vi "Write_Parameter_To_Data_Packet.vi"(8 "error in (no error)":errorcluster, 10 "Parameter value":string, 11 "Parameter name":string) -> (0 "error out":errorcluster, 3 "Data Packets Out":T1[](array[typedef]))   [LabVIEW 2017]
uses:
  Controls/Data Packets/Data_Packet.ctl
  Controls/Packet/Packet.ctl
  Controls/Packet/Packet_Direction.ctl
  Controls/Packet/Packet_Type.ctl
  Controls/Packet/Packet_Priority.ctl
  Controls/Data Packets/Parameter.ctl
  Controls/Data Packets/Parameter_Data_Type.ctl
  Controls/Data Packets/Data_Packet_Transmit_Mode.ctl
  Controls/Data Packets/Data_Packet_FGV_Commands.ctl
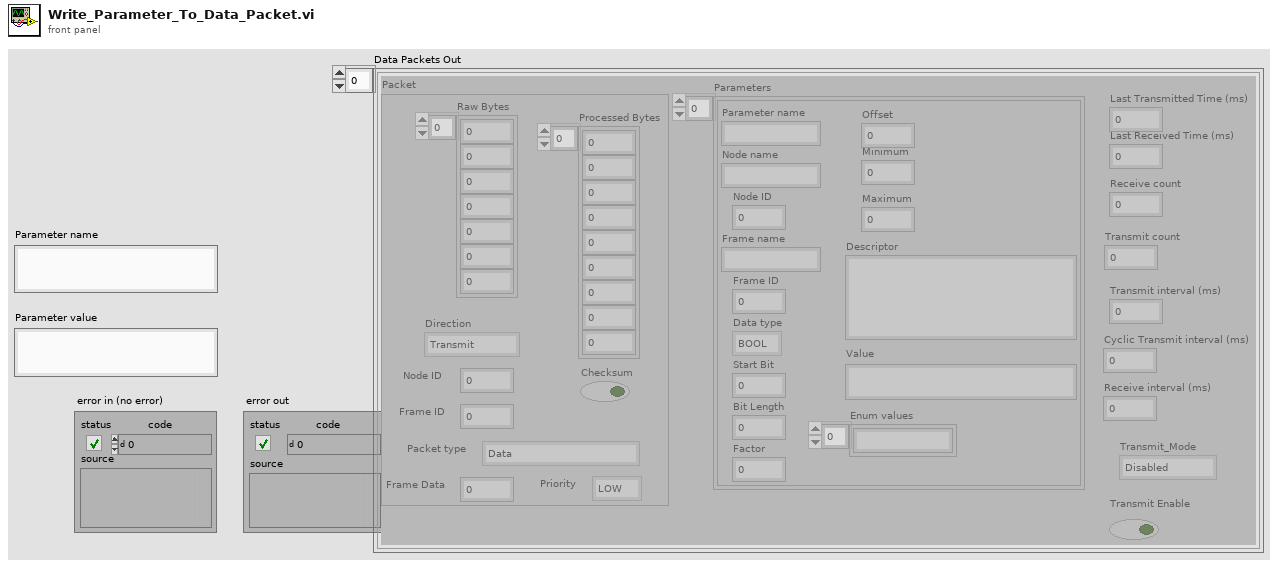
[diagram p1: front panel]
types:
  T1 = typedef "Data_Packet.ctl" = cluster{"Packet":T2, "Parameters":T6[], "Last Received Time (ms)":u64, "Receive count":i32, "Transmit count":i32, "Transmit interval (ms)":u32, "Last Transmitted Time (ms)":u64, "Receive interval (ms)":u32, "Transmit_Mode":T8, "Transmit Enable":bool, "Cyclic Transmit interval (ms)":u32}
  T2 = typedef "Packet.ctl" = cluster{"Raw Bytes":u8[], "Checksum":bool, "Direction":T3, "Processed Bytes":u8[], "Node ID":u8, "Packet type":T4, "Frame Data":u32, "Priority":T5, "Frame ID":u8}
  T3 = typedef "Packet_Direction.ctl" = enum16{"Transmit", "Receive", "Bidirectional"}
  T4 = typedef "Packet_Type.ctl" = enum16{"Data", "Connection Management", "Remote Request", "Error/Status"}
  T5 = typedef "Packet_Priority.ctl" = enum16{"LOW", "HIGH"}
  T6 = typedef "Parameter.ctl" = cluster{"Parameter name":string, "Node name":string, "Node ID":u8, "Frame name":string, "Frame ID":u8, "Data type":T7, "Start Bit":i32, "Bit Length":i32, "Factor":dbl, "Offset":dbl, "Minimum":dbl, "Maximum":dbl, "Descriptor":string, "Enum values":string[], "Value":string}
  T7 = typedef "Parameter_Data_Type.ctl" = enum16{"BOOL", "UNSIGNED", "SIGNED", "FLOAT32", "ENUM"}
  T8 = typedef "Data_Packet_Transmit_Mode.ctl" = enum16{"Disabled", "Single", "Cyclic"}
  T9 = typedef "Data_Packet_FGV_Commands.ctl" = enum16{"Update all parameters from data packets", "Update Packet", "Load", "Read Packet Parameters", "Write Packet Parameters", "Read Packet Parameter", "Write Packet Parameter", "Read Data Packets", "Read Data Packet", "Read Data Packet by Parameter Name", "Get Parameter Node and Frame ID", "Read Data Packet from Node ID and Frame ID"}
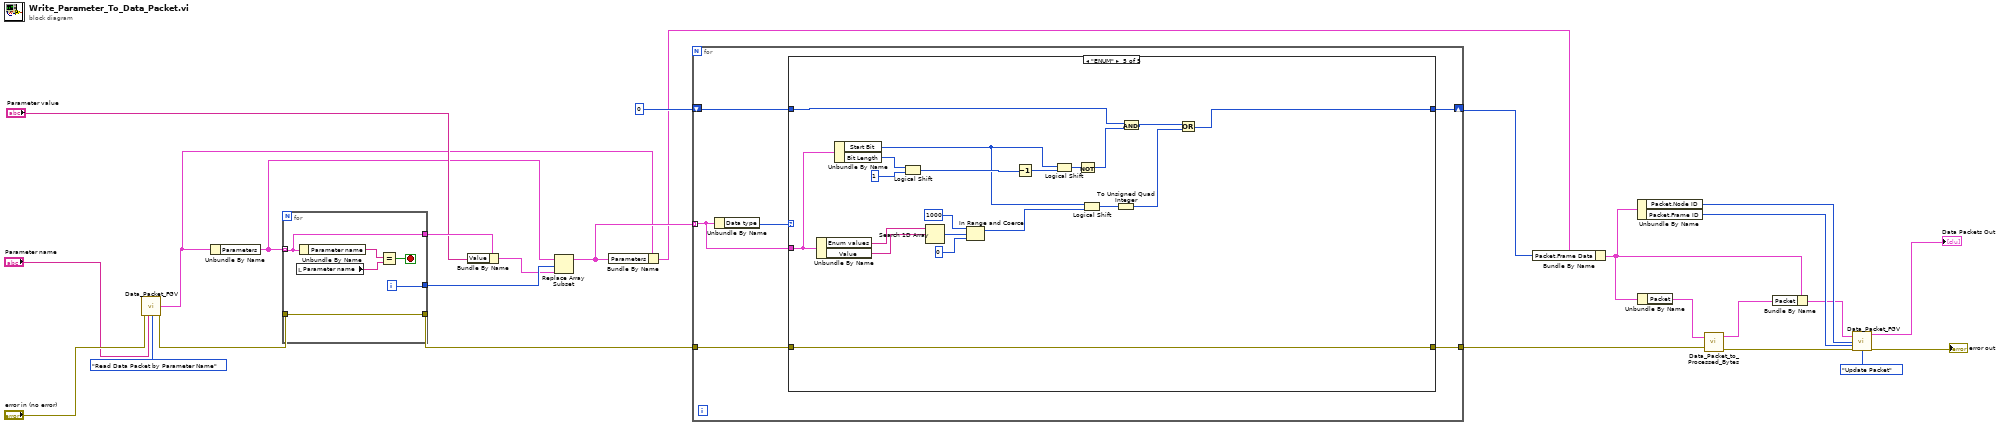
[diagram p0: block diagram]
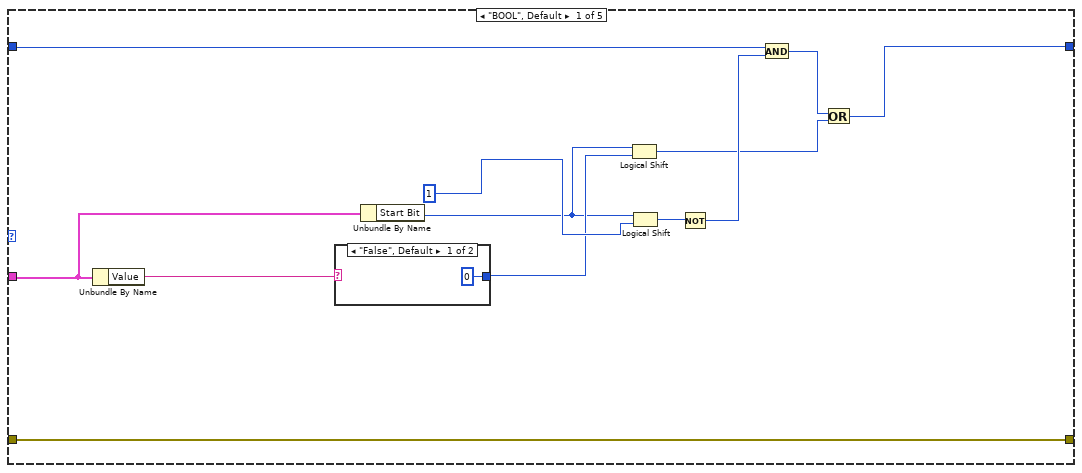
[diagram p2: hidden frame]
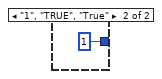
[diagram p3: hidden frame]
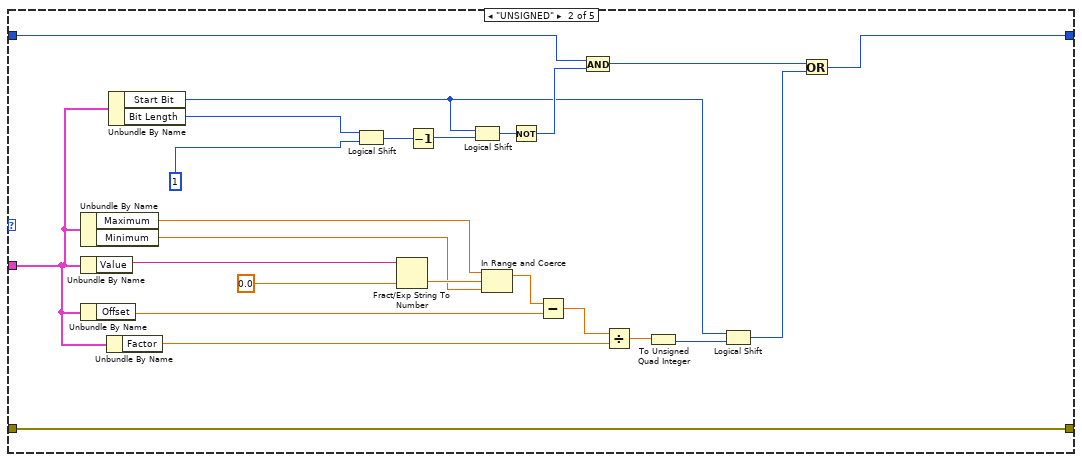
[diagram p4: hidden frame]
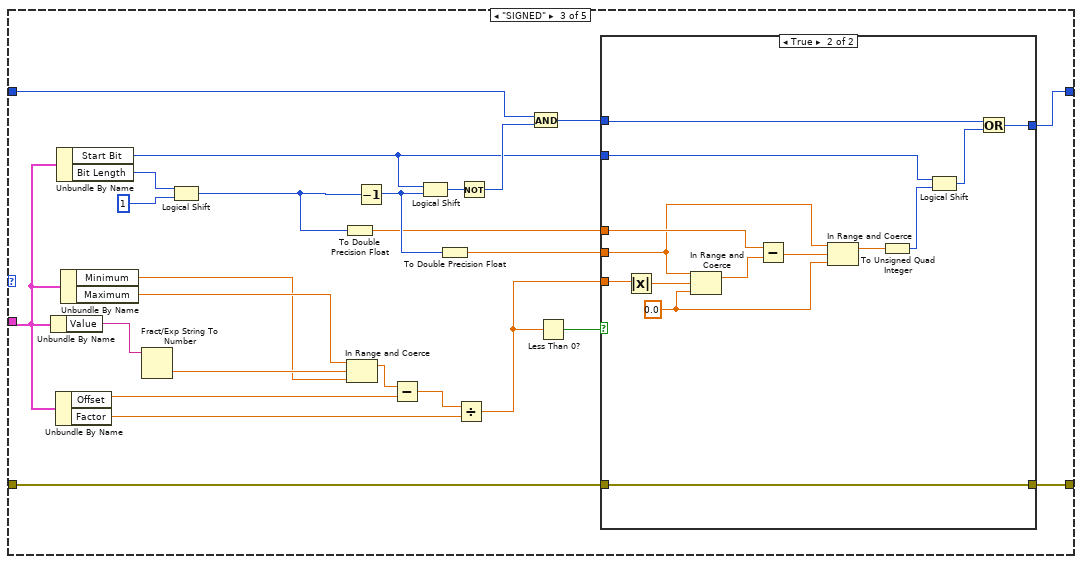
[diagram p5: hidden frame]
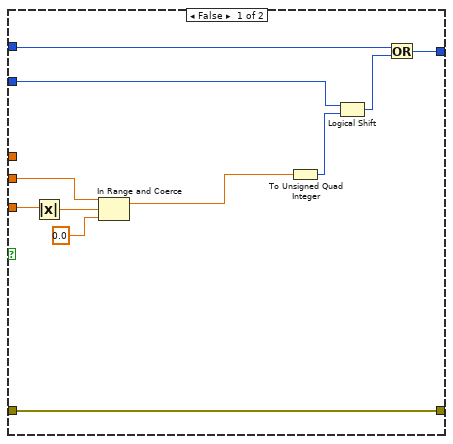
[diagram p6: hidden frame]
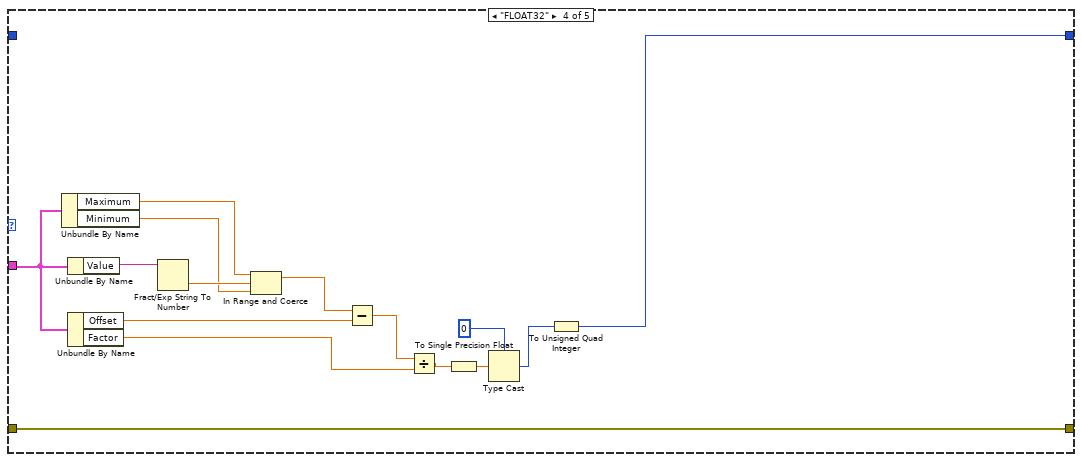
[diagram p7: hidden frame]
diagram:
  n1 = call "Data_Packet_FGV.vi"("error in (no error)"="error in (no error)", "Parameter name"="Parameter name", "Commands"=Data_Packet_FGV_Commands."Read Data Packet by Parameter Name") -> ("Data_Packet out"=w2:T1, "error out"=w23:errorcluster)  [unwired: 7 in, 4 out]
  n2 = Unbundle By Name(w2) -> ("Parameters"=w20:T6[])
  n3 = for {
    tunnel: w23 -> [w27]
    tunnel: w20 -> [w28] mode=indexing
    tunnel: [w30] -> w19
    tunnel: [w28] -> w22
    tunnel: [w27] -> w17
    i -> [w30]
    stop <- w29 stop-if-true
    n4 = local read "Parameter name"() -> (w31:string)
    n5 = Unbundle By Name(w28) -> ("Parameter name"=w32:string)
    n6 = Equal?(x=w32, y=w31) -> (x = y?=w29:bool)
  }
  n7 = Bundle By Name(cluster=w22, "Value"="Parameter value") -> (w18:T6)
  n8 = Replace Array Subset(array=w20, new element=w18, index=w19) -> (w16:T6[])
  n9 = Bundle By Name(cluster=w2, "Parameters"=w16) -> (w1:T1)
  n10 = for {
    tunnel: w17 -> [w38]
    tunnel: w16 -> [w35] mode=indexing
    shift-right: [w34] -> w14
    shift-left: u64 0 -> [w36]
    tunnel: [w33] -> w12
    n11 = Unbundle By Name(w35) -> ("Data type"=w37:T7)
    n12 = case shown="\"ENUM\"" w37 {
      tunnel: w38 -> [w39 w67 w78 w127 w143]
      tunnel: w36 -> [w46 w60 w93 _ w151]
      tunnel: w35 -> [w49 w65 w90 w137 w150]
      tunnel: [w40 w53 w79 w128 w144] -> w34
      tunnel: [w39 w67 w77 w127 w143] -> w33
      frame "BOOL", Default {
        n13 = Unbundle By Name(w49) -> ("Value"=w50:string)
        n14 = case shown="\"False\", Default" w50 {
          tunnel: [u64 0 u64 1] -> w44
          frame "False", Default {
          }
          frame "1", "TRUE", "True" {
          }
        }
        n15 = Unbundle By Name(w49) -> ("Start Bit"=w43:i32)
        n16 = Logical Shift(y=w43, x=w44) -> (x << y=w41:u64)
        n17 = Logical Shift(y=w43, x=u64 1) -> (x << y=w47:u64)
        n18 = Not(x=w47) -> (.not. x?=w45:u64)
        n19 = And(x=w46, y=w45) -> (x .and. y?=w42:u64)
        n20 = Or(x=w42, y=w41) -> (x .or. y?=w40:u64)
      }
      frame "UNSIGNED" {
        n21 = Unbundle By Name(w65) -> ("Maximum"=w71:dbl, "Minimum"=w70:dbl)
        n22 = Unbundle By Name(w65) -> ("Value"=w76:string)
        n23 = Unbundle By Name(w65) -> ("Offset"=w74:dbl)
        n24 = Unbundle By Name(w65) -> ("Factor"=w68:dbl)
        n25 = Unbundle By Name(w65) -> ("Start Bit"=w55:i32, "Bit Length"=w64:i32)
        n26 = Logical Shift(y=w64, x=u64 1) -> (x << y=w62:u64)
        n27 = Fract/Exp String To Number(string=w76, default (0 dbl)=0.0 ("default (0 DBL)")) -> (number=w72:dbl)  [unwired: 2 in, 1 out]
        n28 = Decrement(x=w62) -> (x-1=w61:u64)
        n29 = Logical Shift(y=w55, x=w61) -> (x << y=w59:u64)
        n30 = In Range and Coerce(upper limit=w71, x=w72, lower limit=w70) -> (coerced(x)=w69:dbl)  [unwired: 1 out]
        n31 = Not(x=w59) -> (.not. x?=w58:u64)
        n32 = Subtract(x=w69, y=w74) -> (x-y=w73:dbl)
        n33 = And(x=w60, y=w58) -> (x .and. y?=w57:u64)
        n34 = Divide(x=w73, y=w68) -> (x/y=w66:dbl)
        n35 = To Unsigned Quad Integer(1:w66) -> (0:w56:u64)
        n36 = Logical Shift(y=w55, x=w56) -> (x << y=w54:u64)
        n37 = Or(x=w57, y=w54) -> (x .or. y?=w53:u64)
      }
      frame "SIGNED" {
        n38 = Unbundle By Name(w90) -> ("Value"=w101:string)
        n39 = Unbundle By Name(w90) -> ("Offset"=w100:dbl, "Factor"=w98:dbl)
        n40 = Unbundle By Name(w90) -> ("Start Bit"=w80:i32, "Bit Length"=w97:i32)
        n41 = Unbundle By Name(w90) -> ("Minimum"=w88:dbl, "Maximum"=w89:dbl)
        n42 = Fract/Exp String To Number(string=w101) -> (number=w91:dbl)  [unwired: 3 in, 1 out]
        n43 = Logical Shift(y=w97, x=u64 1) -> (x << y=w83:u64)
        n44 = To Double Precision Float(number=w83) -> (double precision float=w82:dbl)
        n45 = In Range and Coerce(upper limit=w89, x=w91, lower limit=w88) -> (coerced(x)=w92:dbl)  [unwired: 1 out]
        n46 = Decrement(x=w83) -> (x-1=w85:u64)
        n47 = Subtract(x=w92, y=w100) -> (x-y=w99:dbl)
        n48 = Logical Shift(y=w80, x=w85) -> (x << y=w95:u64)
        n49 = To Double Precision Float(number=w85) -> (double precision float=w84:dbl)
        n50 = Divide(x=w99, y=w98) -> (x/y=w86:dbl)
        n51 = Not(x=w95) -> (.not. x?=w94:u64)
        n52 = And(x=w93, y=w94) -> (x .and. y?=w81:u64)
        n53 = Less Than 0?(x=w86) -> (x < 0?=w87:bool)
        n54 = case shown="True" w87 {
          tunnel: w86 -> [w112 w126]
          tunnel: w84 -> [w110 w121]
          tunnel: w82 -> [_ w124]
          tunnel: w81 -> [w106 w116]
          tunnel: w80 -> [w107 w117]
          tunnel: [w104 w114] -> w79
          tunnel: w78 -> [w102 w113]
          tunnel: [w102 w113] -> w77
          frame False {
            n55 = Absolute Value(x=w112) -> (abs(x)=w111:dbl)
            n56 = In Range and Coerce(upper limit=w110, x=w111, lower limit=0.0) -> (coerced(x)=w103:dbl)  [unwired: 1 out]
            n57 = To Unsigned Quad Integer(1:w103) -> (0:w108:u64)
            n58 = Logical Shift(y=w107, x=w108) -> (x << y=w105:u64)
            n59 = Or(x=w106, y=w105) -> (x .or. y?=w104:u64)
          }
          frame True {
            w120 = 0.0 ("lower limit")
            n60 = Absolute Value(x=w126) -> (abs(x)=w125:dbl)
            n61 = In Range and Coerce(upper limit=w121, x=w125, lower limit=w120) -> (coerced(x)=w123:dbl)  [unwired: 1 out]
            n62 = Subtract(x=w124, y=w123) -> (x-y=w122:dbl)
            n63 = In Range and Coerce(upper limit=w121, x=w122, lower limit=w120) -> (coerced(x)=w119:dbl)  [unwired: 1 out]
            n64 = To Unsigned Quad Integer(1:w119) -> (0:w118:u64)
            n65 = Logical Shift(y=w117, x=w118) -> (x << y=w115:u64)
            n66 = Or(x=w116, y=w115) -> (x .or. y?=w114:u64)
          }
        }
      }
      frame "FLOAT32" {
        n67 = Unbundle By Name(w137) -> ("Maximum"=w135:dbl, "Minimum"=w134:dbl)
        n68 = Unbundle By Name(w137) -> ("Value"=w141:string)
        n69 = Unbundle By Name(w137) -> ("Offset"=w140:dbl, "Factor"=w138:dbl)
        n70 = Fract/Exp String To Number(string=w141) -> (number=w136:dbl)  [unwired: 3 in, 1 out]
        n71 = In Range and Coerce(upper limit=w135, x=w136, lower limit=w134) -> (coerced(x)=w133:dbl)  [unwired: 1 out]
        n72 = Subtract(x=w133, y=w140) -> (x-y=w139:dbl)
        n73 = Divide(x=w139, y=w138) -> (x/y=w132:dbl)
        n74 = To Single Precision Float(number=w132) -> (single precision float=w131:sgl)
        n75 = Type Cast(type=u32 0, x=w131) -> (*(type *) &x=w129:u32)
        n76 = To Unsigned Quad Integer(1:w129) -> (0:w128:u64)
      }
      frame "ENUM" {
        n77 = Unbundle By Name(w150) -> ("Enum values"=w161:string[], "Value"=w160:string)
        n78 = Unbundle By Name(w150) -> ("Start Bit"=w142:i32, "Bit Length"=w148:i32)
        n79 = Logical Shift(y=w148, x=u64 1) -> (x << y=w152:u64)
        n80 = Search 1D Array(1D array=w161, element=w160) -> (index of element=w159:i32)  [unwired: 1 in]
        n81 = In Range and Coerce(upper limit=1000, x=w159, lower limit=0) -> (coerced(x)=w147:i32)  [unwired: 1 out]
        n82 = Decrement(x=w152) -> (x-1=w153:u64)
        n83 = Logical Shift(y=w142, x=w153) -> (x << y=w155:u64)
        n84 = Not(x=w155) -> (.not. x?=w154:u64)
        n85 = Logical Shift(y=w142, x=w147) -> (x << y=w146:i32)
        n86 = To Unsigned Quad Integer(1:w146) -> (0:w145:u64)
        n87 = And(x=w151, y=w154) -> (x .and. y?=w149:u64)
        n88 = Or(x=w149, y=w145) -> (x .or. y?=w144:u64)
      }
    }
  }
  n89 = Bundle By Name(cluster=w1, "Packet.Frame Data"=w14) -> (w9:T1)
  n90 = Unbundle By Name(w9) -> ("Packet.Node ID"=w8:u8, "Packet.Frame ID"=w7:u8)
  n91 = Unbundle By Name(w9) -> ("Packet"=w13:T2)
  n92 = call "Data_Packet_to_Processed_Bytes.vi"("Data Packet In"=w13, "error in (no error)"=w12) -> ("Data Packet Out"=w11:T2, "error out"=w10:errorcluster)  [unwired: 1 out]
  n93 = Bundle By Name(cluster=w9, "Packet"=w11) -> (w5:T1)
  n94 = call "Data_Packet_FGV.vi"("Data_Packet In"=w5, "Node ID"=w8, "Frame ID"=w7, "error in (no error)"=w10, "Commands"=Data_Packet_FGV_Commands."Update Packet") -> ("Data Packets Out"=→"Data Packets Out":T1[], "error out"=→"error out":errorcluster)  [unwired: 5 in, 4 out]
